vi "Compute Peak Density.vi"(8 "error in (no error)":errorcluster, 11 "Video Cam Processor in":refnum<class "Video Cam Processor.lvclass">) -> (0 "error out":errorcluster, 2 "Average Peak Separation Distance":dbl, 3 "Video Cam Processor out":refnum<class "Video Cam Processor.lvclass">)   [LabVIEW 2018, in "Video Cam Processor.lvclass"]
uses:
  Video Cam Processor.lvclass
  Video Cam Processor.lvclass/Video Cam Processor.ctl
  707faa64-82aa-4cb5-90c1-c94426e19f10.vi
  Video Frame/Video Frame.lvclass
  <vilib>/Analysis/NI_AALBase.lvlib
  <vilib>/Analysis/baseanly.llb/Mean (DBL).vi
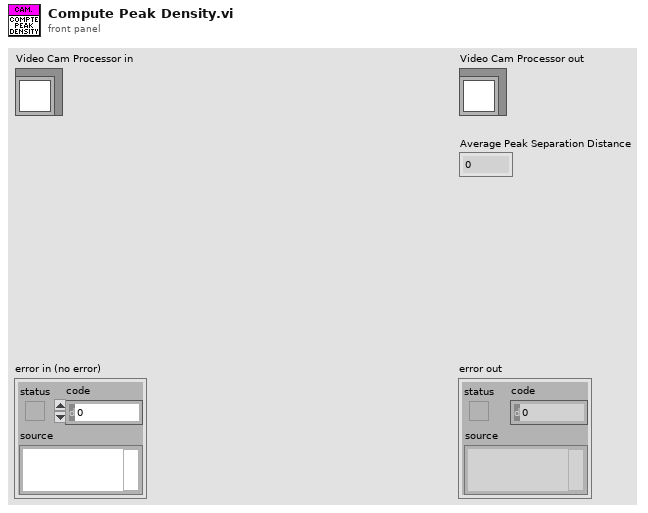
[diagram p1: front panel]
types:
  T1 = typedef "Video Cam Processor.lvclass/Hull Point STYP.ctl" = cluster{"X":i32, "Y":i32}
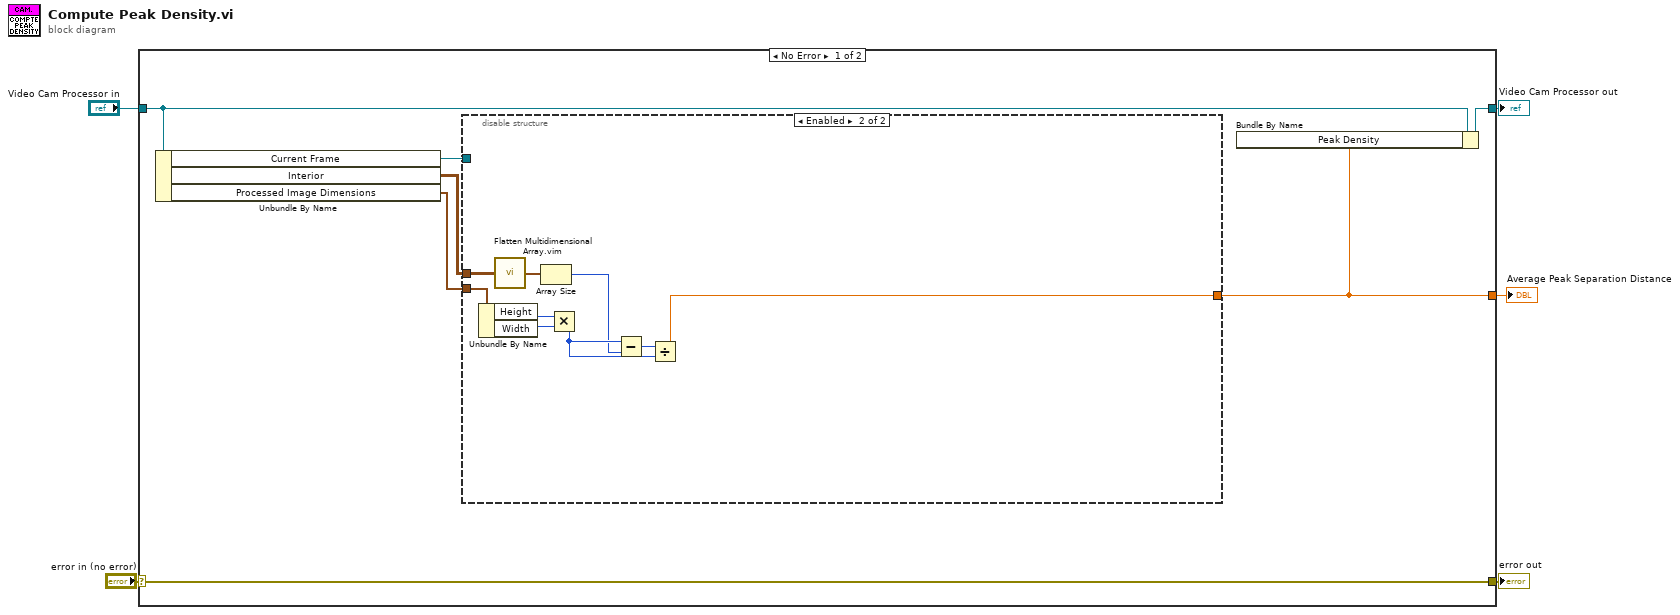
[diagram p0: block diagram]
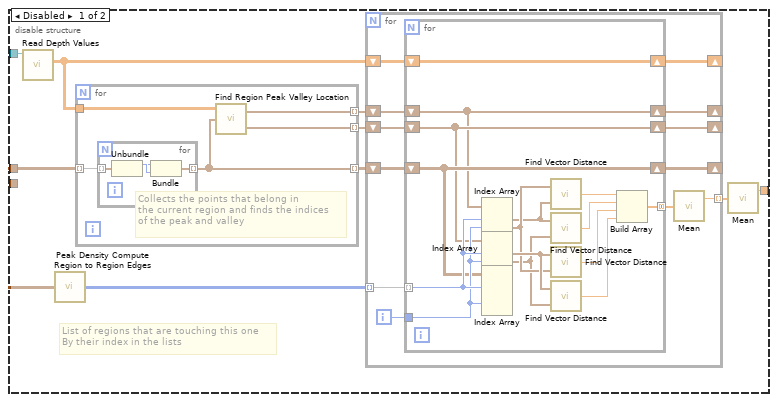
[diagram p2: hidden frame]
diagram:
  n1 = case shown="No Error" "error in (no error)" {
    selector: "error in (no error)" -> [w12 w68]
    tunnel: [w12 w68] -> w4
    tunnel: [w8 w67] -> w2
    tunnel: "Video Cam Processor in" -> [w9 w67]
    tunnel: [w7 _] -> w1
    frame No Error {
      n2 = Unbundle By Name(w9) -> ("Current Frame"=w10:refnum<class "Video Frame.lvclass">, "Interior"=w11:T1[][], "Processed Image Dimensions"=w6:cluster{"Height":i32, "Width":i32})
      n3 = disable-structure shown="Enabled" {
        disable-tunnel: w11 -> [w21 w60]
        disable-tunnel: w10 -> [w16 _]
        disable-tunnel: [w13 w61] -> w7
        disable-tunnel: w6 -> [_ w66]
        frame Disabled {
          # "List of regions that are touching this one\nBy their index in the lists"
          n4 = call-dynamic "Read Depth Values.vi"("Video Frame in"=w16) -> ("Depth Values"=w15:dbl[][])  [unwired: 8 in, 2 out]
          n5 = call "Peak Density Compute Region to Region Edges.vi"("All Regions"=w21) -> ("Edges"=w20:i32[][])
          n6 = for {
            tunnel: w21 -> [w53] mode=indexing
            tunnel: [w52] -> w19 mode=indexing
            tunnel: [w51] -> w18 mode=indexing
            tunnel: [w50] -> w17 mode=indexing
            tunnel: w15 -> [w49]
            # "Collects the points that belong in\nthe current region and finds the indices\nof the peak and valley"
            n7 = for {
              tunnel: w53 -> [w57] mode=indexing
              tunnel: [w54] -> w52 mode=indexing
              n8 = Unbundle(w57) -> ("X"=w56:i32, "Y"=w55:i32)
              n9 = Bundle("Y"=w55, "X"=w56) -> (w54:cluster{"Y":i32, "X":i32})  [unwired: 1 in]
            }
            n10 = call "Find Region Peak Valley Location.vi"("Region Points"=w52, "Depth Values"=w49) -> ("Valley Point Location"=w50:cluster{"Y":i32, "X":i32}, "Peak Point Location"=w51:cluster{"Y":i32, "X":i32})  [unwired: 1 in]
          }
          n11 = for {
            tunnel: w20 -> [w33] mode=indexing
            shift-right: [w31] -> _
            shift-left: w19 -> [w32]
            shift-right: [w28] -> _
            shift-left: w18 -> [w30]
            shift-right: [w27] -> _
            shift-left: w17 -> [w29]
            shift-right: [w24] -> _
            shift-left: w15 -> [w25]
            tunnel: [w22] -> w14 mode=indexing
            i -> [w26]
            n12 = for {
              tunnel: w33 -> [w47] mode=indexing
              shift-right: [w45] -> w31
              shift-left: w32 -> [w45]
              shift-right: [w43] -> w28
              shift-left: w30 -> [w43]
              shift-right: [w44] -> w27
              shift-left: w29 -> [w44]
              tunnel: w26 -> [w46]
              shift-right: [w48] -> w24
              shift-left: w25 -> [w48]
              tunnel: [w34] -> w23 mode=concatenating
              n13 = Index Array(array=w43, index #1=w47, index #2=w46) -> (element #1=w40:cluster{"Y":i32, "X":i32}, element #2=w41:cluster{"Y":i32, "X":i32})
              n14 = Index Array(array=w44, index #1=w47, index #2=w46) -> (element #1=w42:cluster{"Y":i32, "X":i32}, element #2=w39:cluster{"Y":i32, "X":i32})
              n15 = Index Array(array=w45, index (row) #1=w47, index (row) #2=w46) -> ()  [unwired: 2 in, 2 out]
              n16 = call "Find Vector Distance.vi"("Point B"=w40, "Point A"=w41) -> ("Distance Between A and B"=w38:dbl)
              n17 = call "Find Vector Distance.vi"("Point B"=w39, "Point A"=w40) -> ("Distance Between A and B"=w37:dbl)
              n18 = call "Find Vector Distance.vi"("Point B"=w41, "Point A"=w42) -> ("Distance Between A and B"=w36:dbl)
              n19 = call "Find Vector Distance.vi"("Point B"=w39, "Point A"=w42) -> ("Distance Between A and B"=w35:dbl)
              n20 = Build Array(w38, w37, w36, w35) -> (w34:dbl[])
            }
            n21 = call-poly <vilib>:"Mean.vi"("X"=w23) -> ("mean"=w22:dbl)  [unwired: 1 out]
          }
          n22 = call-poly <vilib>:"Mean.vi"("X"=w14) -> ("mean"=w13:dbl)  [unwired: 1 out]
        }
        frame Enabled {
          n23 = Unbundle By Name(w66) -> ("Height"=w64:i32, "Width"=w65:i32)
          n24 = call "Flatten Multidimensional Array.vim"("Array"=w60) -> ("output array"=w59:T1[])  [unwired: 14 in]
          n25 = Array Size(array=w59) -> (size(s)=w58:i32)
          n26 = Multiply(x=w64, y=w65) -> (x*y=w62:i32)
          n27 = Subtract(x=w62, y=w58) -> (x-y=w63:i32)
          n28 = Divide(x=w63, y=w62) -> (x/y=w61:dbl)
        }
      }
      n29 = Bundle By Name(cluster=w9, "Peak Density"=w7) -> (w8:refnum<class "Video Cam Processor.lvclass">)
    }
    frame Error {
    }
  }
  "error out" <- w4
  "Video Cam Processor out" <- w2
  "Average Peak Separation Distance" <- w1
